vi "Waveform and Laser Controls V7.vi"() -> ()   [LabVIEW 2014]
uses:
  Waveform Scan Parameters.ctl
  <vilib>/Platform/TimedLoop/XDataNode/timing_clust.ctl
  <vilib>/Platform/TimedLoop/XDataNode/nitl_modes.ctl
  <vilib>/Platform/TimedLoop/XDataNode/wakeup.ctl
  <vilib>/rvi/Emulation/niFpgaGetClockAttributes.vi
  <vilib>/rvi/Emulation/niFpgaSctlEmulationGetInTimedLoop.vi
  <vilib>/rvi/Emulation/niFpgaEmulationReportErrorSimple.vi
  <vilib>/rvi/Emulation/niFpgaProcessEmulError.vi
  <vilib>/rvi/eio/common/nirviEmuTemplateMethod_errors.vi
  <vilib>/rvi/Emulation/niFpgaCriticalErrorInLSC.vi
  <vilib>/rvi/Memory/Memory_Emulation/nirvimemoryFastEmulation.vi
  <vilib>/rvi/Memory/Memory_Emulation/nirvimemoryEmulation.vi
  <vilib>/rvi/Emulation/niFpgaEmulationIsFPGAContextNoSignature.vi
  <vilib>/rvi/DataTransferAndStorage/Container/Common/niFpgaContainerGetUniqueNameForEmu.vi
  <vilib>/rvi/errors/nirviReportUnexpectedCaseInternalError (U32).vi
  <vilib>/rvi/Memory/Memory_Emulation/niFpgaMemoryEmulationCacheClearOnFirstRun.vi
  <vilib>/rvi/Memory/Memory_Emulation/nirvimemoryEmulationManagerCache_MakeExclusive.vi
  <vilib>/rvi/Memory/Memory_Emulation/niFpgaMemoryEmulationValidateCache.vi
  <vilib>/rvi/Memory/Memory_Emulation/nirvimemoryEmulationManagerCache_InsertValue.vi
  <vilib>/Utility/error.llb/Clear Errors.vi
  <vilib>/rvi/Memory/Memory_Emulation/nirvimemoryEmulationManagerCache_ReleaseExclusive.vi
  <vilib>/rvi/Memory/Memory_Emulation/nirvimemoryEmulationManagerCache_GetValue.vi
  <vilib>/rvi/Memory/Memory_Emulation/nirvimemoryEmulationManagerCache_SetValue.vi
  <vilib>/eio/EIONode/EIONode.xnode
  <vilib>/rvi/DataTransferAndStorage/Container/XNode/niFpgaContainer.xnode
  <vilib>/Platform/TimedLoop/XDataNode/XDataNode.xnode
  <vilib>/rvi/DataTransferAndStorage/Register/Emulation/niFpgaRegisterEmulation.vi
  <vilib>/Platform/TimedLoop/XDataNode/XDNodeRunTimeDep.lvlib
panel:
  in  "Current Frame":u8
  in  "Lower Shutter Command":bool
  in  "Upper Shutter Command":bool
  out "Lower Shutter Status":bool
  out "Upper Shutter Status":bool
  in  "stop":bool
  in  "775 AOM (I16)":i16=16500
  out "Laser Blank Trigger":bool
  in  "Laser On Time (Ticks)":u8=8
  in  "Sequences":u8=4
  in  "Laser Delay (Ticks)":u8
  in  "Laser States":u32
  in  "Blanking Off/Manual":bool
  in  "Z Piezo Axis":i16
  in  "Y Piezo Axis":i16
  in  "X Piezo Axis":i16
  out "End Linear Ramp":bool
  in  "End of Linear Ramp":u32
  in  "Z Stack Start Position (I16)":i16
  in  "Frames Per Z Step":u8
  in  "Number of Z Steps":u8
  in  "Z Step Size (I16)":i16
  in  "Stop Sync Signal":bool
  in  "Accums Per Line":u32[](array[numeric])=[0, 0, 0, 0]
  in  "Number of Lines":u32
  out "Frame Trigger":bool
  in  "Reset Position Error":bool
  in  "Galvo 1 Position (I16)":i16
  in  "Galvo 2 Position (I16)":i16
  in  "WF 3 Data Loaded":bool
  in  "WF 2 Data Loaded":bool
  in  "Waveform Scan Parameters":T1={"Scanning Mode"=0, "Fast Axis WF Length (Elements)"=0, "Fast Axis Sample Period (Ticks)"=40, "Slow Axis 1 WF Length (Elements)"=0, "Slow Axis 1 Sample Period (Ticks)"=40, "Slow Axis 1 Delay (25 ns) Steps"=40, "Slow Axis 2 WFLength (Elements)"=0, "Slow Axis 2 Sample Period (Ticks)"=40, "Slow Axis 2 Delay (25 ns) Steps"=40}
  in  "Resonant Mirror":T2
  in  "Galvo Mirror 2":T3
  in  "Galvo Mirror 1":T3
  in  "Start Waveforms":bool
  in  "Unused Axis Offset":i16
  in  "Slow Axis 2 Waveform Element":i16
  in  "Fast Axis Waveform Element":i16
  in  "Slow Axis 1 Waveform Element":i16
  in  "WF 1 Data Loaded":bool
  # "V2 - Adding in a line clock\nV3 - Cluster Scan Parameters"
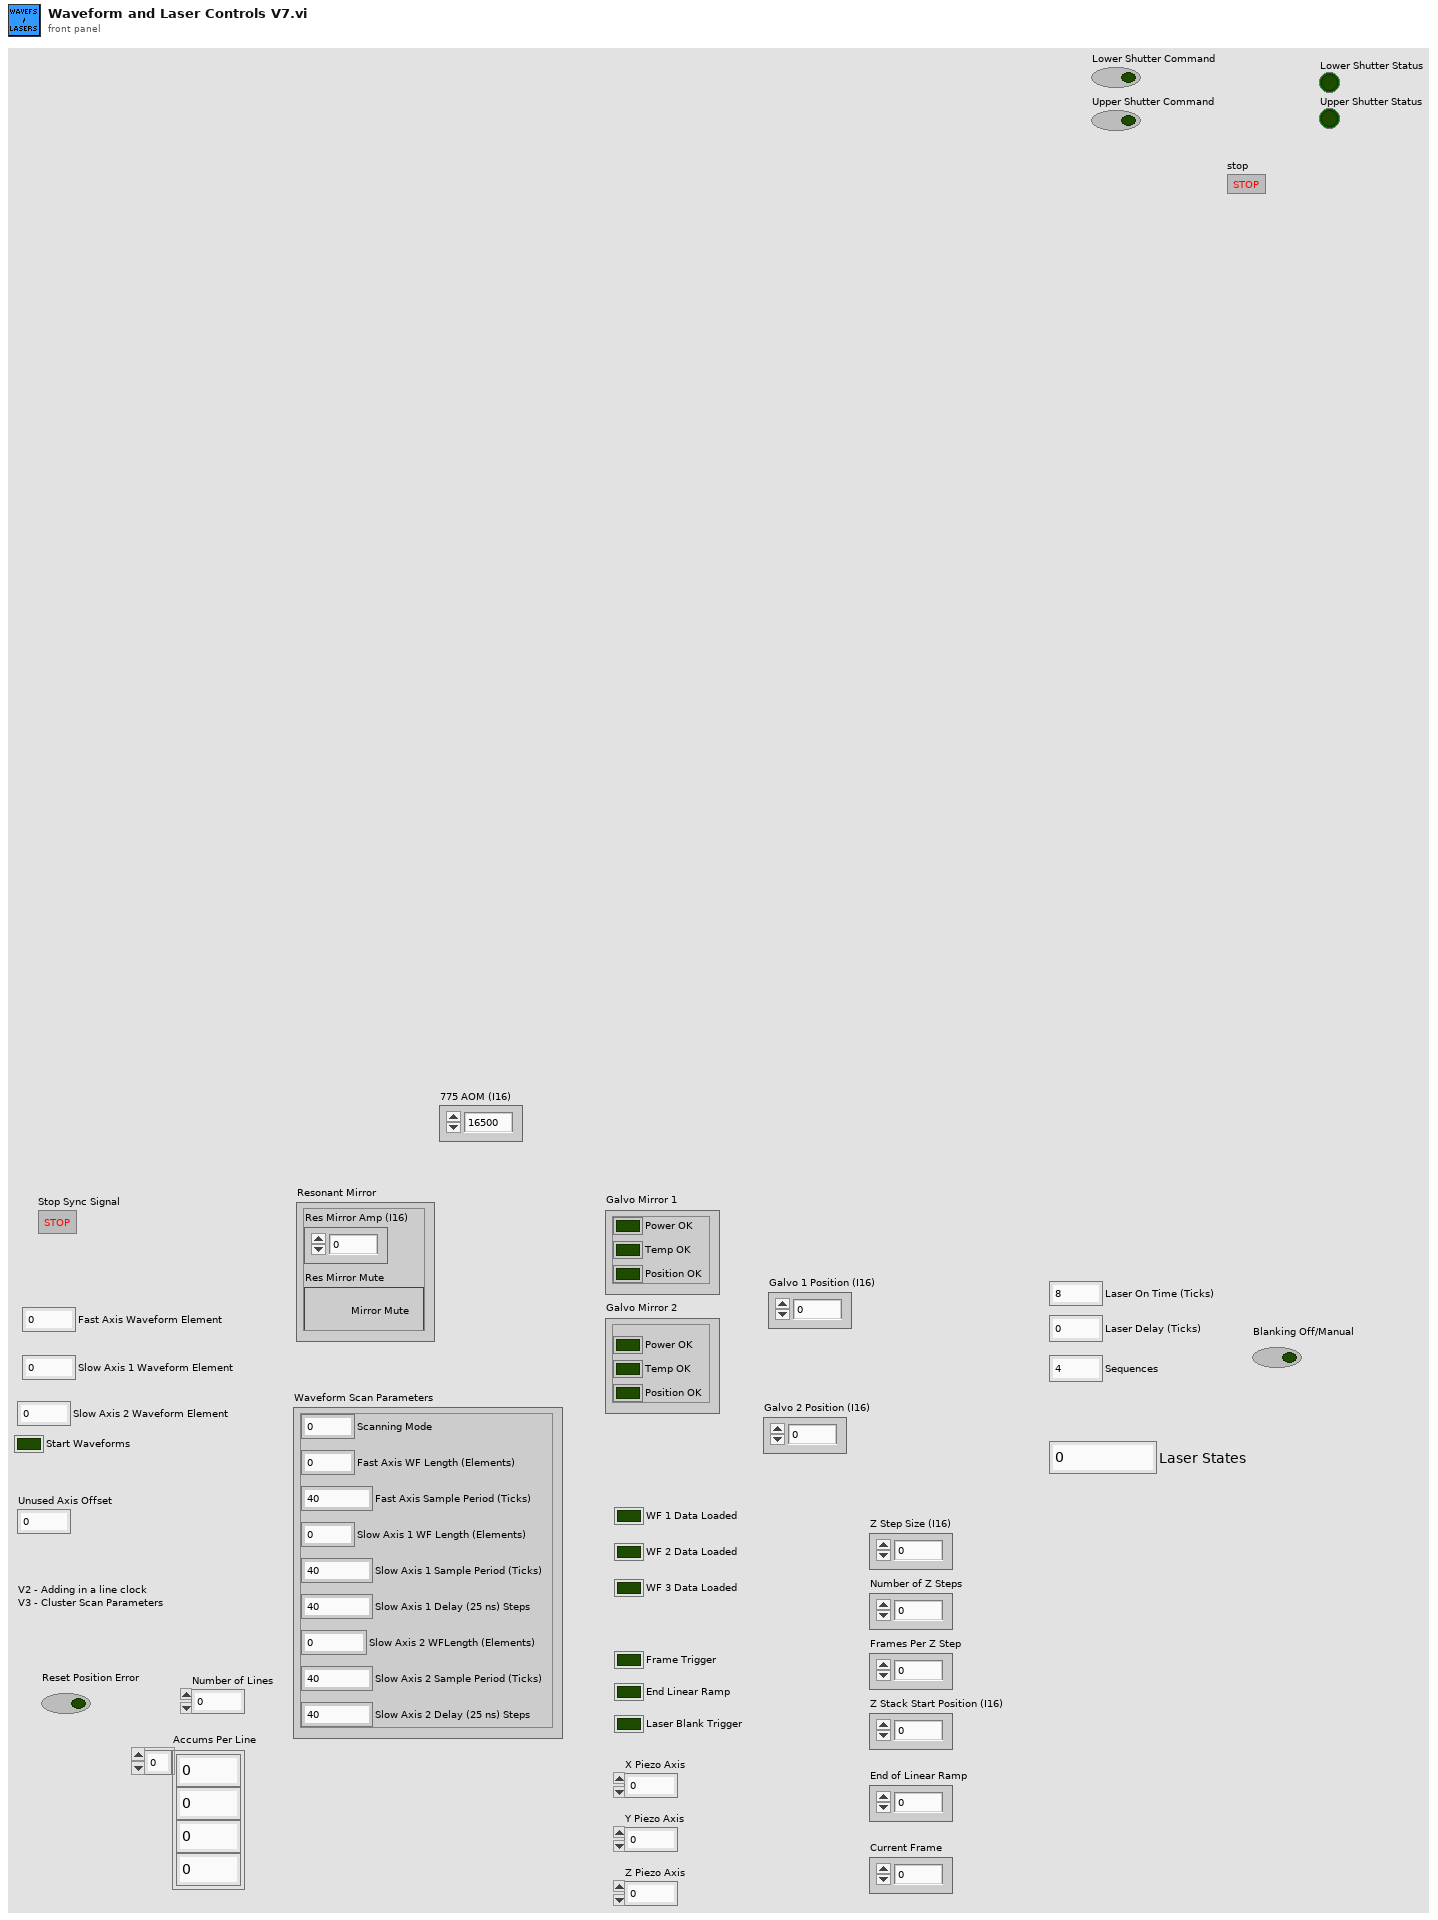
[diagram p1: front panel]
types:
  T1 = typedef "Waveform Scan Parameters.ctl" = cluster{"Scanning Mode":u8, "Fast Axis WF Length (Elements)":i32, "Fast Axis Sample Period (Ticks)":u32, "Slow Axis 1 WF Length (Elements)":i32, "Slow Axis 1 Sample Period (Ticks)":u32, "Slow Axis 1 Delay (25 ns) Steps":i32, "Slow Axis 2 WFLength (Elements)":i32, "Slow Axis 2 Sample Period (Ticks)":u32, "Slow Axis 2 Delay (25 ns) Steps":i32}
  T2 = cluster{"Res Mirror Amp (I16)":i16, "Res Mirror Mute":bool}
  T3 = cluster{"Power OK":bool, "Temp OK":bool, "Position OK":bool}
  T4 = typedef "XDNodeRunTimeDep.lvlib/timing_clust.ctl" = cluster{"Expected End [f-1]":u64, "Actual End [f-1]":u64, "Finished Late? [f-1]":bool, "Expected End [i-1]":u64, "Actual End [i-1]":u64, "Finished Late? [i-1]":bool, "Expected Start [i]":u64, "Actual Start [i]":u64, "Expected Start [f]":u64, "Actual Start [f]":u64, "Source Name":string, "Structure Name":string, "Period":i64, "Deadline":i64, "Offset":i64, "Start":i64, "Priority":i32, "Timeout":i32, "Mode":T5, "Wakeup Reason":T6, "Error":errorcluster, "Source Type":string, "Secondary Source Type":string, "Global End Time":u64, "Global Start Time":u64, "Frame Duration":u64, "Iteration Duration":u64, "Assigned CPU":i32, "I/O Scan Engine Mode":u32}
  T5 = typedef "XDNodeRunTimeDep.lvlib/nitl_modes.ctl" = enum32{"No Change", "Process missed periods, maintain original phase", "Discard missed periods, maintain original phase", "Process missed periods, ignore original phase", "Discard missed periods, ignore original phase"}
  T6 = typedef "XDNodeRunTimeDep.lvlib/wakeup.ctl" = enum32{"Normal", "Aborted", "Asynchronous wakeup", "Timing source error", "Timed loop error", "Timeout"}
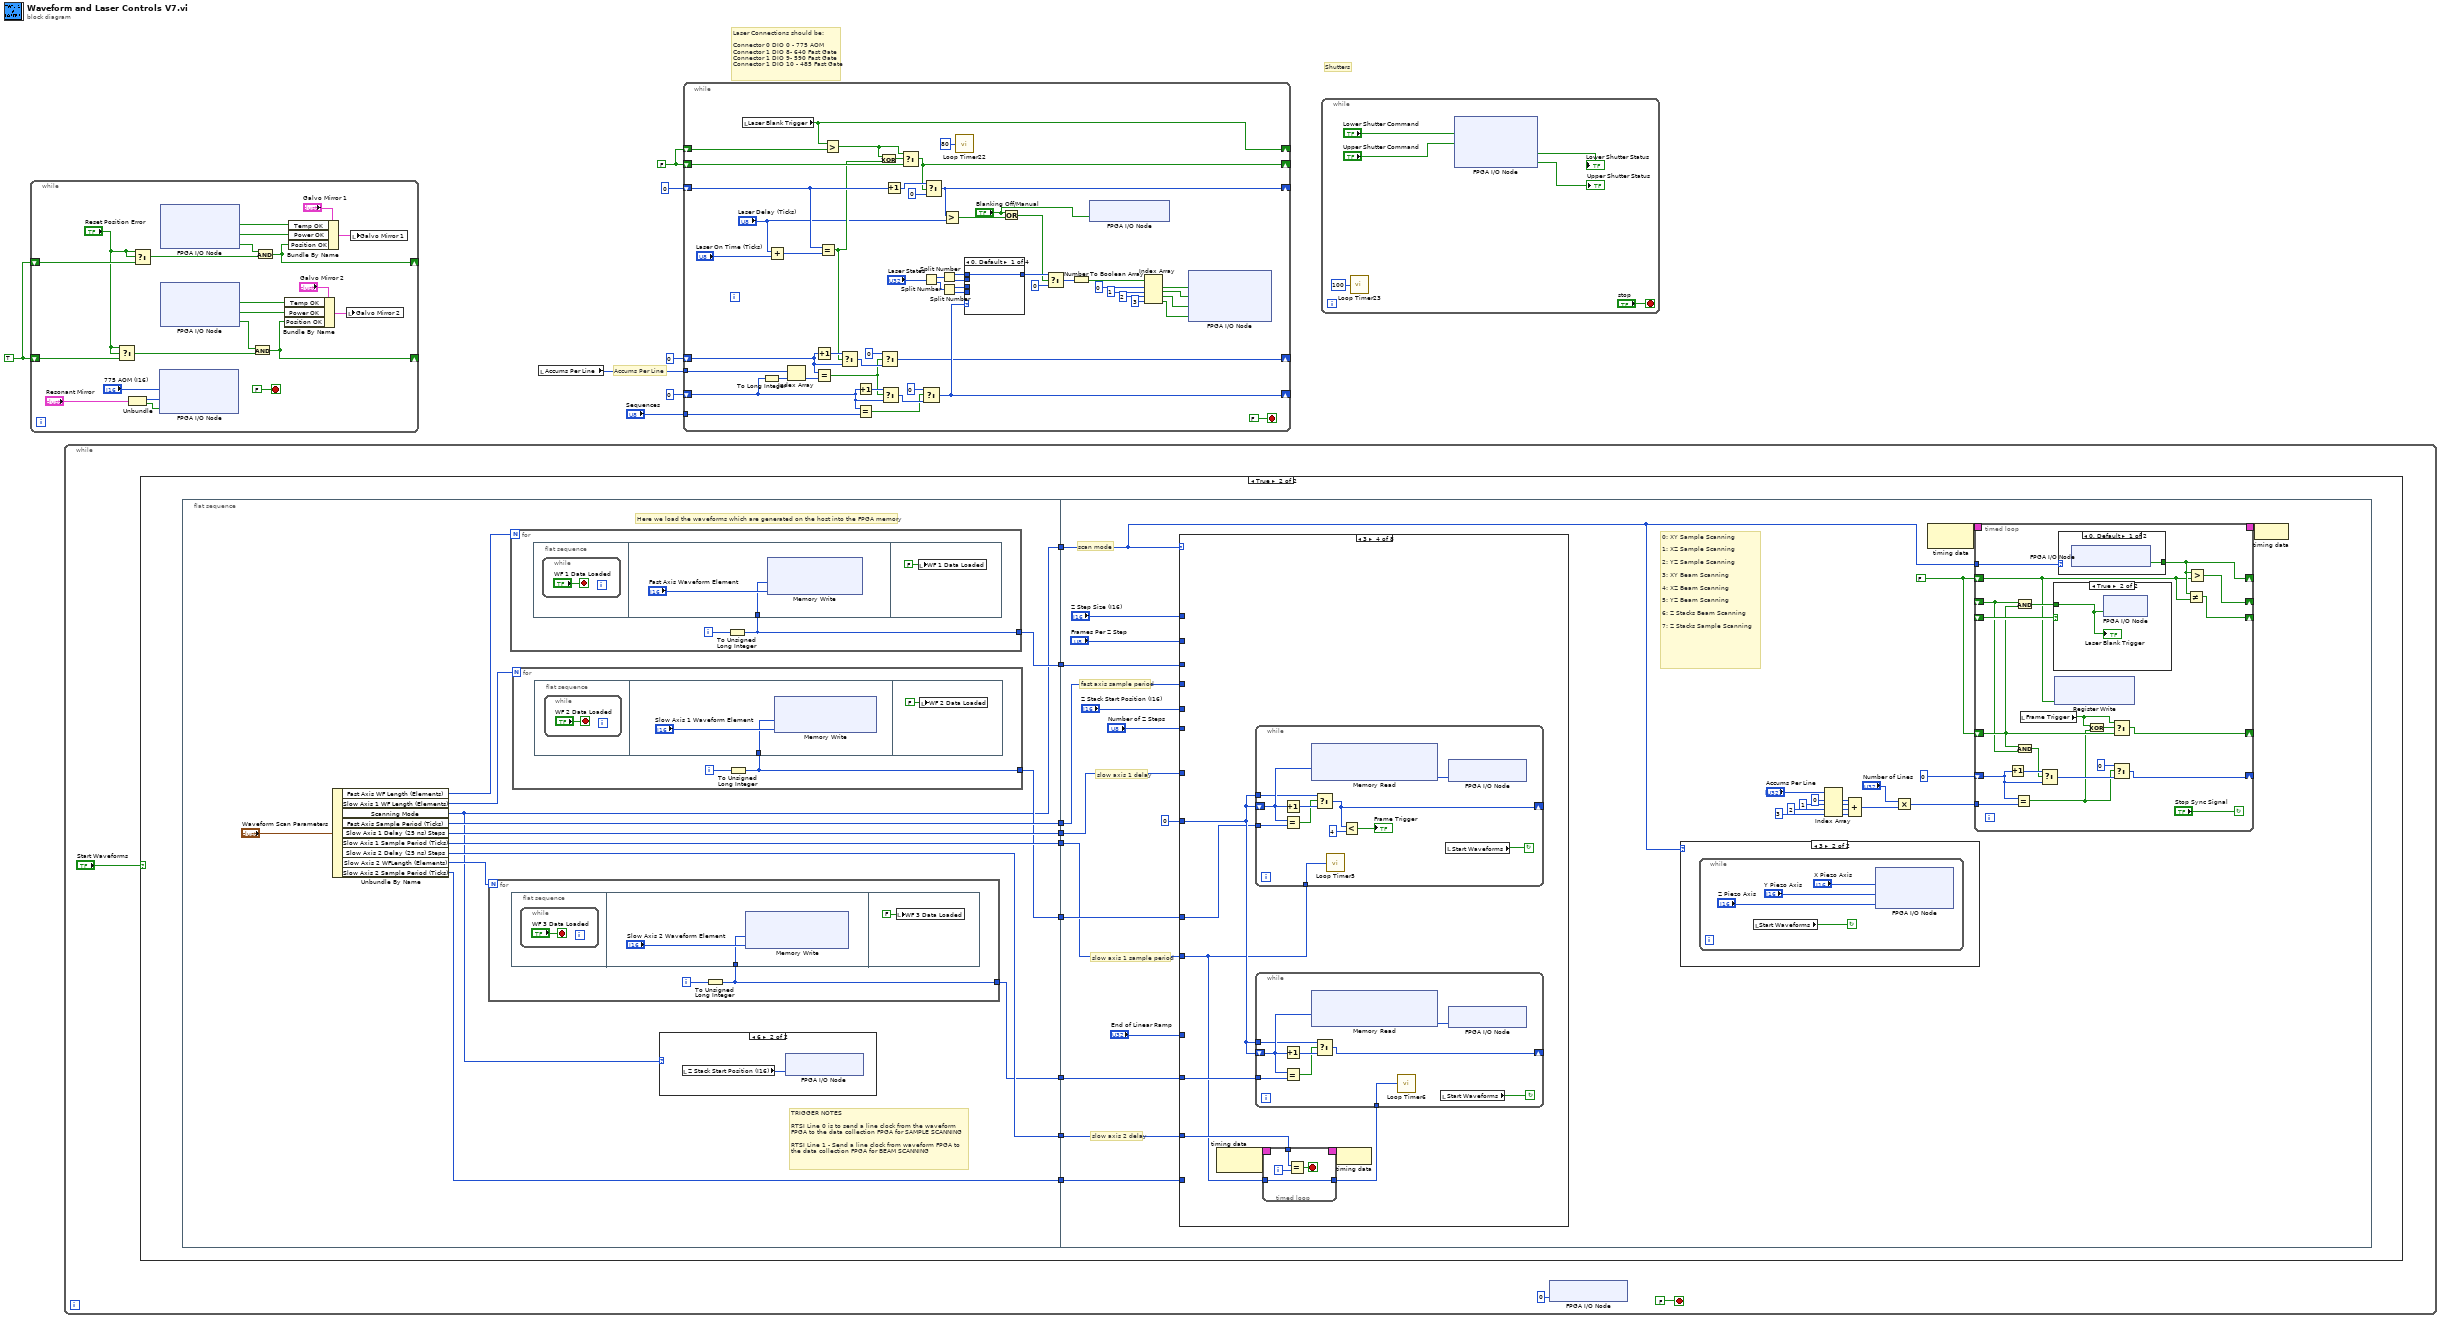
[diagram p0: block diagram]
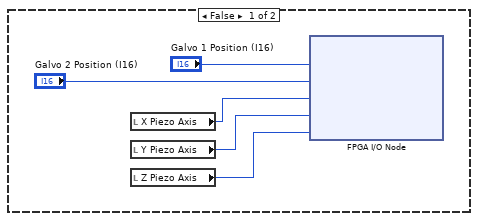
[diagram p5: hidden frame]
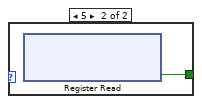
[diagram p7: hidden frame]
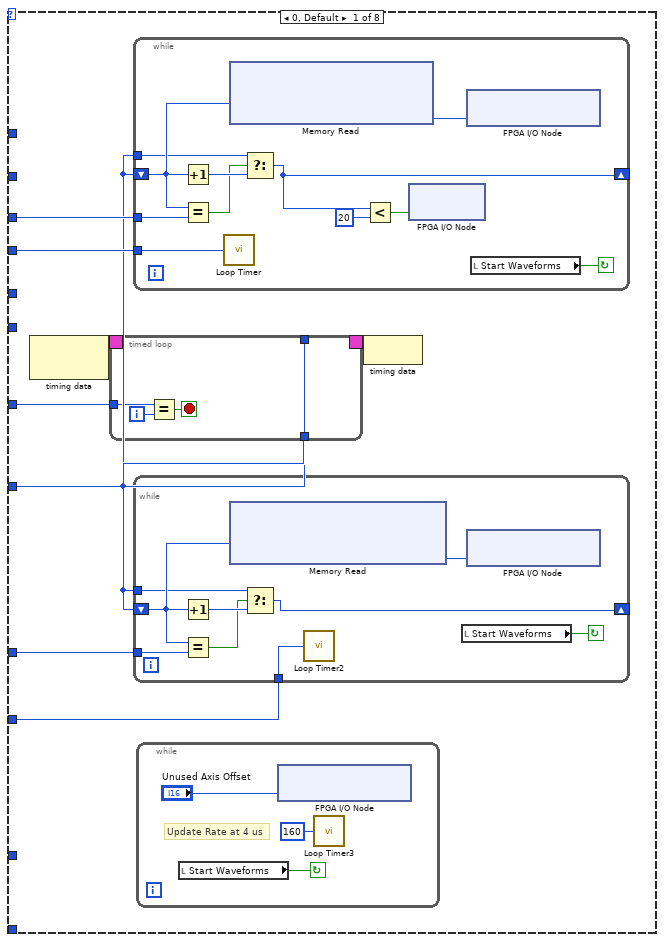
[diagram p10: hidden frame]
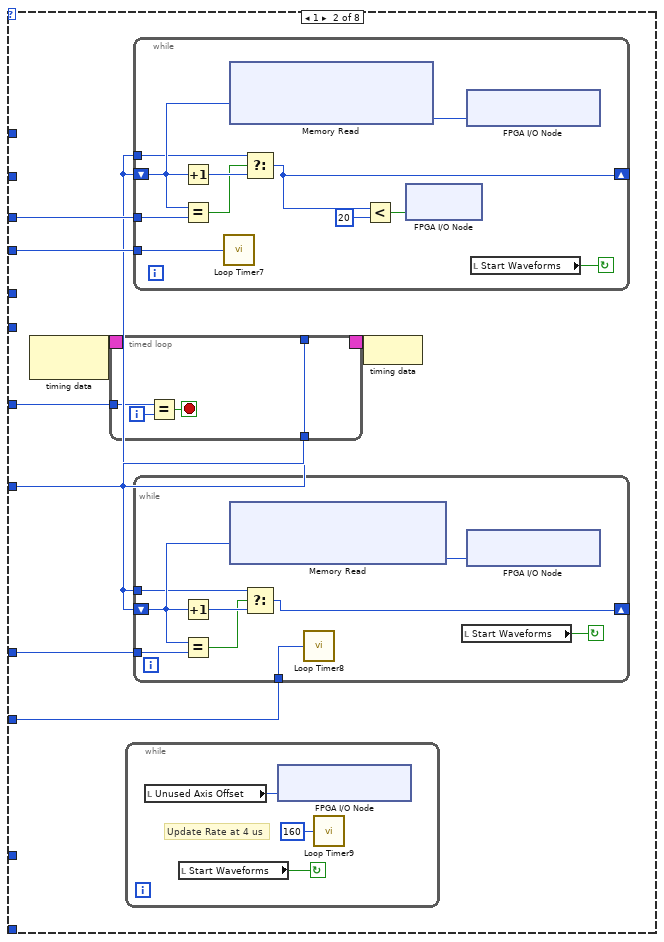
[diagram p11: hidden frame]
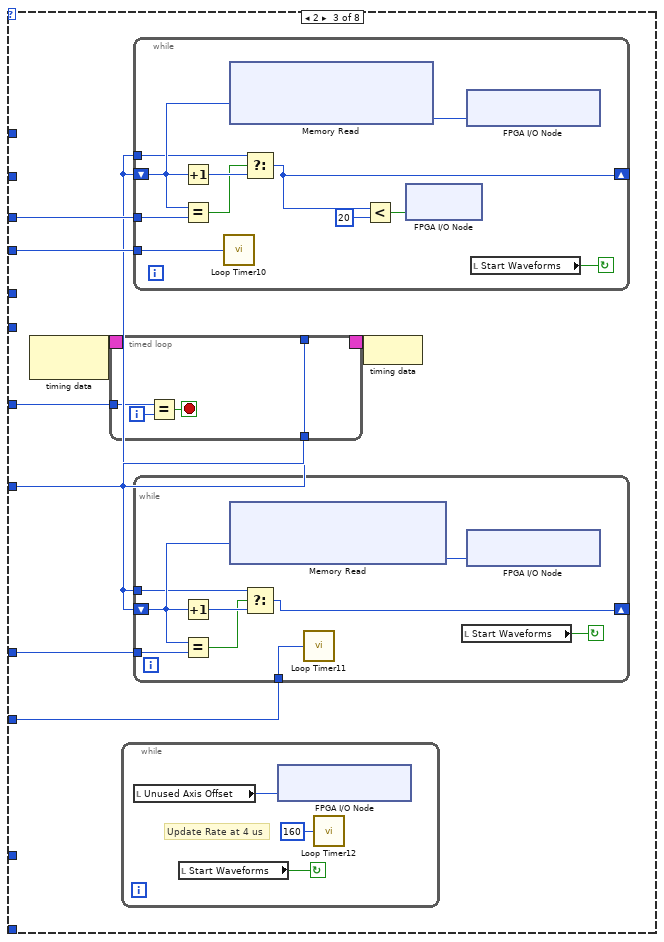
[diagram p12: hidden frame]
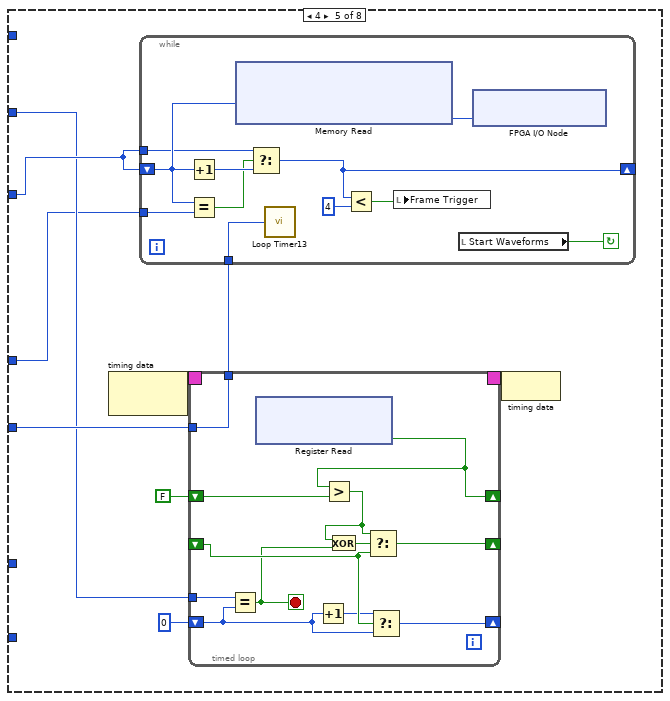
[diagram p13: hidden frame]
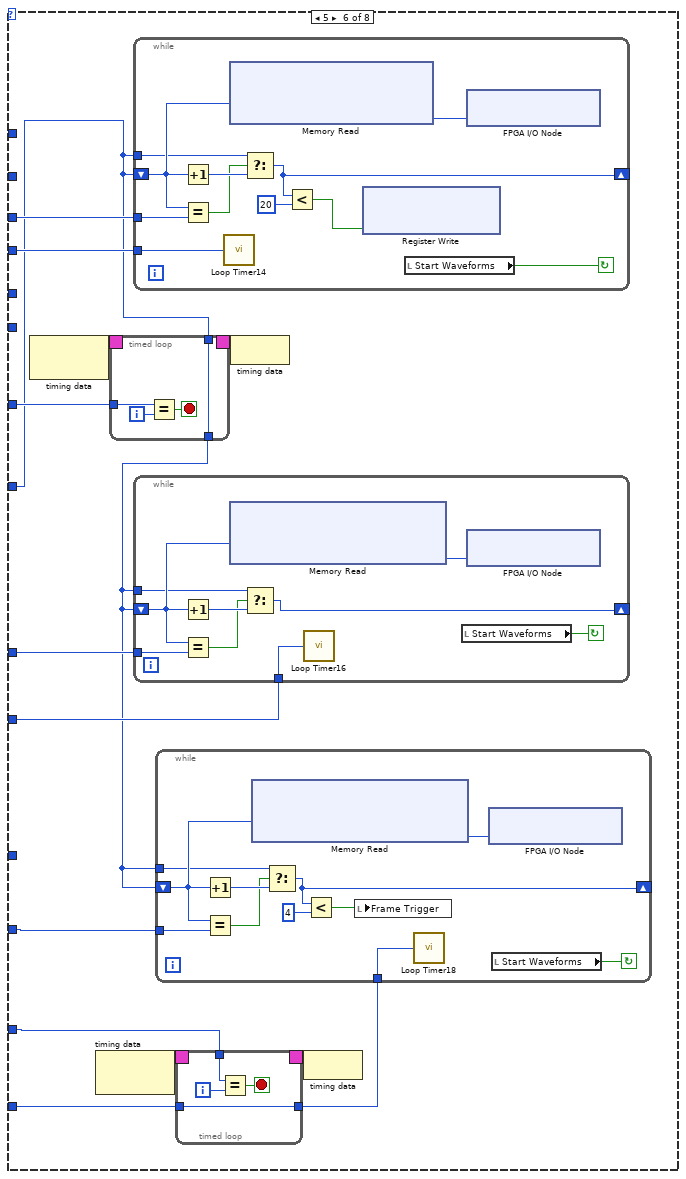
[diagram p14: hidden frame]
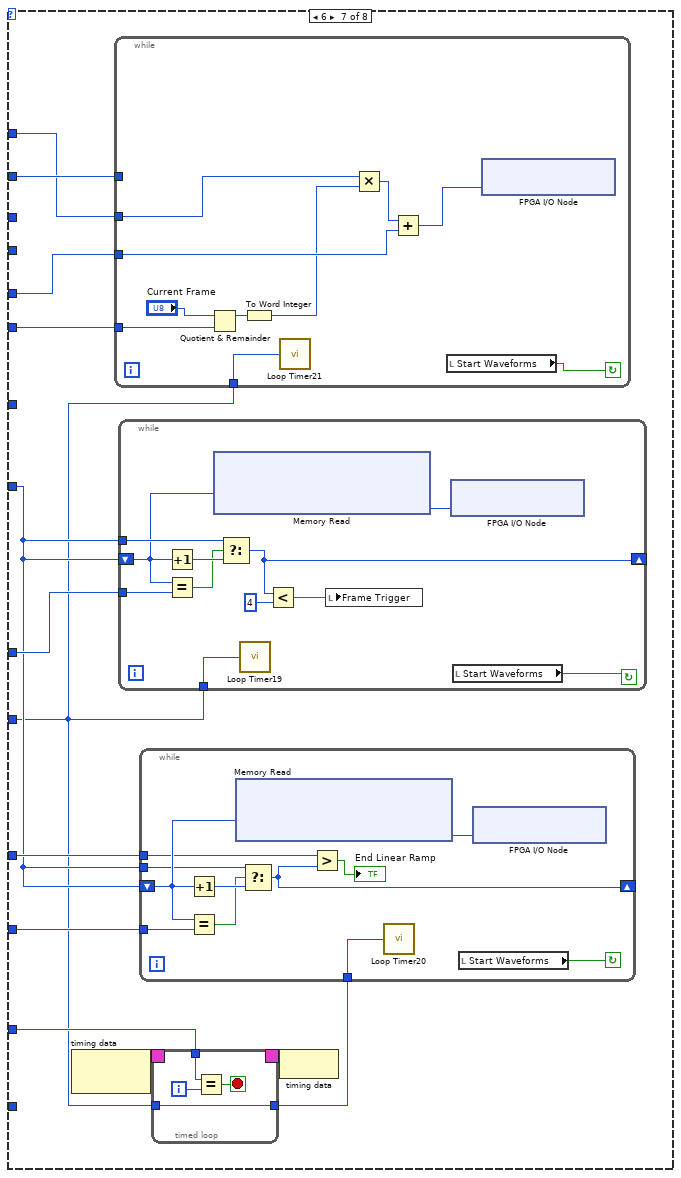
[diagram p15: hidden frame]
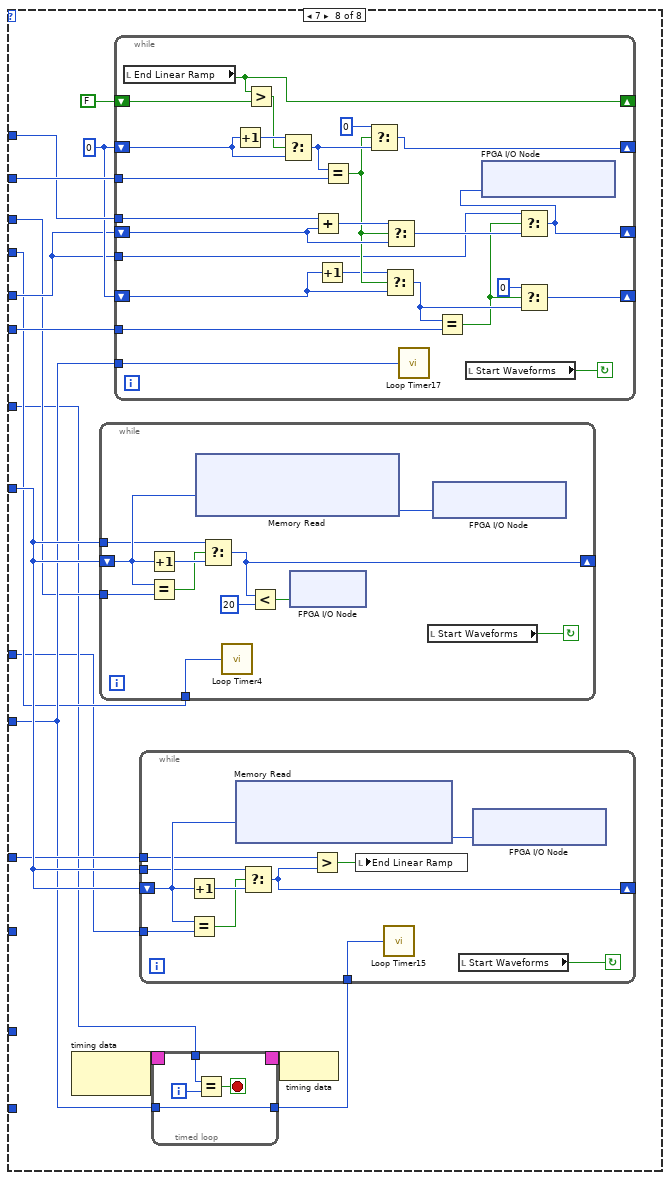
[diagram p16: hidden frame]
diagram:
  w2 = FALSE
  w7 = TRUE
  # "Shutters"
  # "Laser Connections should be:\n\nConnector 0 DIO 0 - 775 AOM\nConnector 1 DIO 8- 640 Fast Gate\nConnector 1 DIO 9- 590 Fast Gate\nConnector 1 DIO 10 - 485 Fast Gate"
  # "Accums Per Line"
  n1 = while {
    shift-right: [w15] -> _
    shift-left: w7 -> [w17]
    shift-right: [w11] -> _
    shift-left: w7 -> [w13]
    stop <- FALSE stop-if-true
    n2 = Select(t="Reset Position Error", s="Reset Position Error", f=w17) -> (s? t:f=w16:bool)
    n3 = Unbundle("Resonant Mirror") -> ("Res Mirror Amp (I16)"=w27:i16, "Res Mirror Mute"=w26:bool)
    n4 = Select(t="Reset Position Error", s="Reset Position Error", f=w13) -> (s? t:f=w12:bool)
    n5 = xnode "FPGA I/O Node"("Connector0/AO4"="775 AOM (I16)", "Connector0/AO7"=w27, "Connector0/DIO7"=w26) -> ()  [unwired: 4 in, 4 out]
    n6 = xnode "FPGA I/O Node"() -> ("Connector0/DIO1"=w8:bool, "Connector0/DIO2"=w25:bool, "Connector0/DIO3"=w14:bool)  [unwired: 4 in, 4 out]
    n7 = xnode "FPGA I/O Node"() -> ("Connector0/DIO4"=w19:bool, "Connector0/DIO5"=w20:bool, "Connector0/DIO6"=w18:bool)  [unwired: 4 in, 4 out]
    n8 = And(x=w18, y=w16) -> (x .and. y?=w15:bool)
    n9 = And(x=w14, y=w12) -> (x .and. y?=w11:bool)
    n10 = Bundle By Name(cluster="Galvo Mirror 2", "Temp OK"=w19, "Power OK"=w20, "Position OK"=w15) -> (w22:T3)
    n11 = Bundle By Name(cluster="Galvo Mirror 1", "Temp OK"=w8, "Power OK"=w25, "Position OK"=w11) -> (w24:T3)
    n12 = local write "Galvo Mirror 2"(w22) -> ()
    n13 = local write "Galvo Mirror 1"(w24) -> ()
  }
  n14 = while {
    stop <- FALSE stop-if-true
    n15 = case shown="True" "Start Waveforms" {
      frame False {
        n16 = local read "X Piezo Axis"() -> (w35:i16)
        n17 = local read "Y Piezo Axis"() -> (w34:i16)
        n18 = local read "Z Piezo Axis"() -> (w33:i16)
        n19 = xnode "FPGA I/O Node"("Connector0/AO5"="Galvo 1 Position (I16)", "Connector0/AO6"="Galvo 2 Position (I16)", "Connector0/AO1"=w35, "Connector0/AO2"=w34, "Connector0/AO3"=w33) -> ()  [unwired: 5 in, 5 out]
      }
      frame True {
        n20 = flat-sequence {
          tunnel: [w59] -> w46
          tunnel: [w49] -> w45
          tunnel: [w50] -> w44
          tunnel: [w48] -> w43
          tunnel: [w57] -> w42
          tunnel: [w56] -> w41
          tunnel: [w55] -> w40
          tunnel: [w54] -> w39
          tunnel: [w47] -> w38
          tunnel: w46 -> [w109]
          tunnel: w45 -> [w108]
          tunnel: w44 -> [w106]
          tunnel: w43 -> [w80]
          tunnel: w42 -> [w105]
          tunnel: w41 -> [w104]
          tunnel: w40 -> [w103]
          tunnel: w39 -> [w102]
          tunnel: w38 -> [w79]
          frame #0 {
            # "TRIGGER NOTES\n\nRTSI Line 0 is to send a line clock from the waveform\nFPGA to the data collection FPGA for SAMPLE SCANNING\n\nRTSI Line 1 - Send a line clock from waveform FPGA to\nthe data collection FPGA for BEAM SCANNING"
            # "Here we load the waveforms which are generated on the host into the FPGA memory"
            n21 = Unbundle By Name("Waveform Scan Parameters") -> ("Fast Axis WF Length (Elements)"=w53:i32, "Slow Axis 1 WF Length (Elements)"=w52:i32, "Scanning Mode"=w48:u8, "Fast Axis Sample Period (Ticks)"=w57:u32, "Slow Axis 1 Delay (25 ns) Steps"=w56:i32, "Slow Axis 1 Sample Period (Ticks)"=w55:u32, "Slow Axis 2 Delay (25 ns) Steps"=w54:i32, "Slow Axis 2 WFLength (Elements)"=w51:i32, "Slow Axis 2 Sample Period (Ticks)"=w47:u32)
            n22 = for {
              N: w51 -> [_]
              tunnel: [w61] -> w49
              i -> [w62]
              n23 = flat-sequence {
                tunnel: w61 -> [w64]
                frame #0 {
                  n24 = while {
                    stop <- "WF 3 Data Loaded" stop-if-true
                  }
                }
                frame #1 {
                  n25 = xnode ("Memory Write")("Address"=w64, "Data"="Slow Axis 2 Waveform Element") -> ()  [unwired: 1 in, 1 out]
                }
                frame #2 {
                  n26 = local write "WF 3 Data Loaded"(FALSE ("Host Data Loaded")) -> ()
                }
              }
              n27 = To Unsigned Long Integer(number=w62) -> (unsigned 32bit integer=w61:u32)
            }
            n28 = for {
              N: w53 -> [_]
              tunnel: [w73] -> w59
              i -> [w74]
              n29 = flat-sequence {
                tunnel: w73 -> [w76]
                frame #0 {
                  n30 = while {
                    stop <- "WF 1 Data Loaded" stop-if-true
                  }
                }
                frame #1 {
                  n31 = xnode ("Memory Write")("Address"=w76, "Data"="Fast Axis Waveform Element") -> ()  [unwired: 1 in, 1 out]
                }
                frame #2 {
                  n32 = local write "WF 1 Data Loaded"(FALSE ("Host Data Loaded")) -> ()
                }
              }
              n33 = To Unsigned Long Integer(number=w74) -> (unsigned 32bit integer=w73:u32)
            }
            n34 = for {
              N: w52 -> [_]
              tunnel: [w67] -> w50
              i -> [w68]
              n35 = flat-sequence {
                tunnel: w67 -> [w70]
                frame #0 {
                  n36 = while {
                    stop <- "WF 2 Data Loaded" stop-if-true
                  }
                }
                frame #1 {
                  n37 = xnode ("Memory Write")("Address"=w70, "Data"="Slow Axis 1 Waveform Element") -> ()  [unwired: 1 in, 1 out]
                }
                frame #2 {
                  n38 = local write "WF 2 Data Loaded"(FALSE ("Host Data Loaded")) -> ()
                }
              }
              n39 = To Unsigned Long Integer(number=w68) -> (unsigned 32bit integer=w67:u32)
            }
            n40 = case shown="6" w48 {
              frame 0, Default {
              }
              frame 6 {
                n41 = local read "Z Stack Start Position (I16)"() -> (w60:i16)
                n42 = xnode "FPGA I/O Node"("Connector0/AO3"=w60) -> ()  [unwired: 1 in, 1 out]
              }
            }
          }
          frame #1 {
            w82 = FALSE
            # "slow axis 2 delay"
            # "slow axis 1 sample period"
            # "slow axis 1 delay"
            # "fast axis sample period"
            # "scan mode"
            # "0: XY Sample Scanning\n\n1: XZ Sample Scanning\n\n2: YZ Sample Scanning\n\n3: XY Beam Scanning\n\n4: XZ Beam Scanning\n\n5: YZ Beam Scanning\n\n6: Z Stacks Beam Scanning\n\n7: Z Stacks Sample Scanning"
            n43 = case shown="3" w80 {
              tunnel: w109 -> [w148 w188 w228 _ _ w348 _ w451]
              tunnel: w105 -> [w147 w187 w227 _ _ w347 _ w452]
              tunnel: w108 -> [_ _ _ w269 _ w342 w408 _]
              tunnel: u32 0 -> [w142 w182 w222 w268 w306 w344 w398 w464]
              tunnel: w104 -> [w146 w186 w226 _ w304 w346 _ w450]
              tunnel: w102 -> [_ _ _ w267 _ w341 w407 _]
              tunnel: w106 -> [w144 w184 w224 w262 w303 w345 w404 w449]
              tunnel: w103 -> [w143 w183 w223 w263 w305 w343 w396 w453]
              tunnel: "Frames Per Z Step" -> [_ _ _ _ _ _ w403 w460]
              tunnel: "Z Stack Start Position (I16)" -> [_ _ _ _ _ _ w399 w456]
              tunnel: "Z Step Size (I16)" -> [_ _ _ _ _ _ w402 w459]
              tunnel: "Number of Z Steps" -> [_ _ _ _ _ _ w401 w457]
              tunnel: "End of Linear Ramp" -> [_ _ _ _ _ _ w400 w455]
              tunnel: w79 -> [_ _ _ _ _ w334 _ _]
              frame 0, Default {
                n44 = node-c288() -> (w150:T4)  [unwired: 1 in]
                n45 = timed-loop {
                  timing: w150 -> [_]
                  timing-out: [_] -> w149
                  tunnel: w146 -> [w155]
                  tunnel: w142 -> [w154]
                  tunnel: [w154] -> w145
                  i -> [w157]
                  stop <- w156 stop-if-true
                  n46 = Equal?(x=w155, y=w157) -> (x = y?=w156:bool)
                }
                n47 = while {
                  shift-right: [w173] -> _
                  shift-left: w142 -> [w179]
                  tunnel: w148 -> [w180]
                  tunnel: w147 -> [w177]
                  tunnel: w142 -> [w176]
                  stop <- w175 continue-if-true
                  n48 = Increment(x=w179) -> (x+1=w181:u32)
                  n49 = Equal?(x=w179, y=w180) -> (x = y?=w174:bool)
                  n50 = call "Loop Timer"("Count(Ticks)"=w177) -> ()  [unwired: 1 out]
                  n51 = xnode ("Memory Read")("Address"=w179) -> ("Data"=w178:i16)  [unwired: 1 in, 1 out]
                  n52 = Select(t=w176, s=w174, f=w181) -> (s? t:f=w173:u32)
                  n53 = Less?(x=w173, y=u32 20) -> (x < y?=w171:bool)
                  n54 = xnode "FPGA I/O Node"("TRIG0"=w171) -> ()  [unwired: 1 in, 1 out]
                  n55 = xnode "FPGA I/O Node"("Connector0/AO1"=w178) -> ()  [unwired: 1 in, 1 out]
                  n56 = local read "Start Waveforms"() -> (w175:bool)
                }
                n57 = while {
                  shift-right: [w169] -> _
                  shift-left: w145 -> [w166]
                  tunnel: w144 -> [w168]
                  tunnel: w145 -> [w164]
                  tunnel: w143 -> [w163]
                  stop <- w162 continue-if-true
                  n58 = Increment(x=w166) -> (x+1=w170:u32)
                  n59 = Equal?(x=w166, y=w168) -> (x = y?=w167:bool)
                  n60 = xnode ("Memory Read")("Address"=w166) -> ("Data"=w165:i16)  [unwired: 1 in, 1 out]
                  n61 = Select(t=w164, s=w167, f=w170) -> (s? t:f=w169:u32)
                  n62 = call "Loop Timer2"("Count(Ticks)"=w163) -> ()  [unwired: 1 out]
                  n63 = local read "Start Waveforms"() -> (w162:bool)
                  n64 = xnode "FPGA I/O Node"("Connector0/AO2"=w165) -> ()  [unwired: 1 in, 1 out]
                }
                n65 = while {
                  stop <- w151 continue-if-true
                  # "Update Rate at 4 us"
                  n66 = local read "Start Waveforms"() -> (w151:bool)
                  n67 = xnode "FPGA I/O Node"("Connector0/AO3"="Unused Axis Offset") -> ()  [unwired: 1 in, 1 out]
                  n68 = call "Loop Timer3"("Count(Ticks)"=u32 160) -> ()  [unwired: 1 out]
                }
                n69 = node-c288(w149) -> ()
              }
              frame 1 {
                n70 = node-c288() -> (w190:T4)  [unwired: 1 in]
                n71 = timed-loop {
                  timing: w190 -> [_]
                  timing-out: [_] -> w189
                  tunnel: w186 -> [w195]
                  tunnel: w182 -> [w194]
                  tunnel: [w194] -> w185
                  i -> [w197]
                  stop <- w196 stop-if-true
                  n72 = Equal?(x=w195, y=w197) -> (x = y?=w196:bool)
                }
                n73 = while {
                  stop <- w192 continue-if-true
                  # "Update Rate at 4 us"
                  n74 = local read "Unused Axis Offset"() -> (w191:i16)
                  n75 = local read "Start Waveforms"() -> (w192:bool)
                  n76 = xnode "FPGA I/O Node"("Connector0/AO2"=w191) -> ()  [unwired: 1 in, 1 out]
                  n77 = call "Loop Timer9"("Count(Ticks)"=u32 160) -> ()  [unwired: 1 out]
                }
                n78 = while {
                  shift-right: [w213] -> _
                  shift-left: w182 -> [w219]
                  tunnel: w188 -> [w220]
                  tunnel: w187 -> [w217]
                  tunnel: w182 -> [w216]
                  stop <- w215 continue-if-true
                  n79 = Increment(x=w219) -> (x+1=w221:u32)
                  n80 = Equal?(x=w219, y=w220) -> (x = y?=w214:bool)
                  n81 = call "Loop Timer7"("Count(Ticks)"=w217) -> ()  [unwired: 1 out]
                  n82 = xnode ("Memory Read")("Address"=w219) -> ("Data"=w218:i16)  [unwired: 1 in, 1 out]
                  n83 = Select(t=w216, s=w214, f=w221) -> (s? t:f=w213:u32)
                  n84 = Less?(x=w213, y=u32 20) -> (x < y?=w211:bool)
                  n85 = xnode "FPGA I/O Node"("TRIG0"=w211) -> ()  [unwired: 1 in, 1 out]
                  n86 = xnode "FPGA I/O Node"("Connector0/AO1"=w218) -> ()  [unwired: 1 in, 1 out]
                  n87 = local read "Start Waveforms"() -> (w215:bool)
                }
                n88 = while {
                  shift-right: [w209] -> _
                  shift-left: w185 -> [w206]
                  tunnel: w184 -> [w208]
                  tunnel: w185 -> [w204]
                  tunnel: w183 -> [w203]
                  stop <- w202 continue-if-true
                  n89 = Increment(x=w206) -> (x+1=w210:u32)
                  n90 = Equal?(x=w206, y=w208) -> (x = y?=w207:bool)
                  n91 = xnode ("Memory Read")("Address"=w206) -> ("Data"=w205:i16)  [unwired: 1 in, 1 out]
                  n92 = Select(t=w204, s=w207, f=w210) -> (s? t:f=w209:u32)
                  n93 = call "Loop Timer8"("Count(Ticks)"=w203) -> ()  [unwired: 1 out]
                  n94 = local read "Start Waveforms"() -> (w202:bool)
                  n95 = xnode "FPGA I/O Node"("Connector0/AO3"=w205) -> ()  [unwired: 1 in, 1 out]
                }
                n96 = node-c288(w189) -> ()
              }
              frame 2 {
                n97 = node-c288() -> (w230:T4)  [unwired: 1 in]
                n98 = timed-loop {
                  timing: w230 -> [_]
                  timing-out: [_] -> w229
                  tunnel: w226 -> [w235]
                  tunnel: w222 -> [w234]
                  tunnel: [w234] -> w225
                  i -> [w237]
                  stop <- w236 stop-if-true
                  n99 = Equal?(x=w235, y=w237) -> (x = y?=w236:bool)
                }
                n100 = while {
                  stop <- w232 continue-if-true
                  # "Update Rate at 4 us"
                  n101 = local read "Unused Axis Offset"() -> (w231:i16)
                  n102 = local read "Start Waveforms"() -> (w232:bool)
                  n103 = xnode "FPGA I/O Node"("Connector0/AO1"=w231) -> ()  [unwired: 1 in, 1 out]
                  n104 = call "Loop Timer12"("Count(Ticks)"=u32 160) -> ()  [unwired: 1 out]
                }
                n105 = while {
                  shift-right: [w253] -> _
                  shift-left: w222 -> [w259]
                  tunnel: w228 -> [w260]
                  tunnel: w227 -> [w257]
                  tunnel: w222 -> [w256]
                  stop <- w255 continue-if-true
                  n106 = Increment(x=w259) -> (x+1=w261:u32)
                  n107 = Equal?(x=w259, y=w260) -> (x = y?=w254:bool)
                  n108 = call "Loop Timer10"("Count(Ticks)"=w257) -> ()  [unwired: 1 out]
                  n109 = xnode ("Memory Read")("Address"=w259) -> ("Data"=w258:i16)  [unwired: 1 in, 1 out]
                  n110 = Select(t=w256, s=w254, f=w261) -> (s? t:f=w253:u32)
                  n111 = Less?(x=w253, y=u32 20) -> (x < y?=w251:bool)
                  n112 = xnode "FPGA I/O Node"("TRIG0"=w251) -> ()  [unwired: 1 in, 1 out]
                  n113 = xnode "FPGA I/O Node"("Connector0/AO2"=w258) -> ()  [unwired: 1 in, 1 out]
                  n114 = local read "Start Waveforms"() -> (w255:bool)
                }
                n115 = while {
                  shift-right: [w249] -> _
                  shift-left: w225 -> [w246]
                  tunnel: w224 -> [w248]
                  tunnel: w225 -> [w244]
                  tunnel: w223 -> [w243]
                  stop <- w242 continue-if-true
                  n116 = Increment(x=w246) -> (x+1=w250:u32)
                  n117 = Equal?(x=w246, y=w248) -> (x = y?=w247:bool)
                  n118 = xnode ("Memory Read")("Address"=w246) -> ("Data"=w245:i16)  [unwired: 1 in, 1 out]
                  n119 = Select(t=w244, s=w247, f=w250) -> (s? t:f=w249:u32)
                  n120 = call "Loop Timer11"("Count(Ticks)"=w243) -> ()  [unwired: 1 out]
                  n121 = local read "Start Waveforms"() -> (w242:bool)
                  n122 = xnode "FPGA I/O Node"("Connector0/AO3"=w245) -> ()  [unwired: 1 in, 1 out]
                }
                n123 = node-c288(w229) -> ()
              }
              frame 3 {
                n124 = node-c288() -> (w266:T4)  [unwired: 1 in]
                n125 = while {
                  shift-right: [w289] -> _
                  shift-left: w268 -> [w295]
                  tunnel: w262 -> [w296]
                  tunnel: w263 -> [w293]
                  tunnel: w268 -> [w292]
                  stop <- w291 continue-if-true
                  n126 = Increment(x=w295) -> (x+1=w297:u32)
                  n127 = Equal?(x=w295, y=w296) -> (x = y?=w290:bool)
                  n128 = xnode ("Memory Read")("Address"=w295) -> ("Data"=w294:i16)  [unwired: 1 in, 1 out]
                  n129 = Select(t=w292, s=w290, f=w297) -> (s? t:f=w289:u32)
                  n130 = call "Loop Timer5"("Count(Ticks)"=w293) -> ()  [unwired: 1 out]
                  n131 = Less?(x=w289, y=u32 4) -> (x < y?=→"Frame Trigger":bool)
                  n132 = local read "Start Waveforms"() -> (w291:bool)
                  n133 = xnode "FPGA I/O Node"("Connector0/AO5"=w294) -> ()  [unwired: 1 in, 1 out]
                }
                n134 = timed-loop {
                  timing: w266 -> [_]
                  timing-out: [_] -> w265
                  tunnel: w263 -> [w279]
                  tunnel: [w279] -> w264
                  tunnel: w267 -> [w280]
                  i -> [w282]
                  stop <- w281 stop-if-true
                  n135 = Equal?(x=w280, y=w282) -> (x = y?=w281:bool)
                }
                n136 = while {
                  shift-right: [w277] -> _
                  shift-left: w268 -> [w275]
                  tunnel: w269 -> [w276]
                  tunnel: w264 -> [w273]
                  tunnel: w268 -> [w272]
                  stop <- w271 continue-if-true
                  n137 = Increment(x=w275) -> (x+1=w278:u32)
                  n138 = Equal?(x=w275, y=w276) -> (x = y?=w270:bool)
                  n139 = xnode ("Memory Read")("Address"=w275) -> ("Data"=w274:i16)  [unwired: 1 in, 1 out]
                  n140 = Select(t=w272, s=w270, f=w278) -> (s? t:f=w277:u32)
                  n141 = call "Loop Timer6"("Count(Ticks)"=w273) -> ()  [unwired: 1 out]
                  n142 = local read "Start Waveforms"() -> (w271:bool)
                  n143 = xnode "FPGA I/O Node"("Connector0/AO6"=w274) -> ()  [unwired: 1 in, 1 out]
                }
                n144 = node-c288(w265) -> ()
              }
              frame 4 {
                n145 = node-c288() -> (w301:T4)  [unwired: 1 in]
                n146 = timed-loop {
                  timing: w301 -> [_]
                  timing-out: [_] -> w300
                  tunnel: w305 -> [w309]
                  shift-right: [w307] -> _
                  shift-left: FALSE -> [w318]
                  shift-right: [w315] -> _
                  shift-left: _ -> [w314]
                  shift-right: [w312] -> _
                  shift-left: 0 -> [w310]
                  tunnel: w304 -> [w311]
                  tunnel: [w309] -> w302
                  stop <- w308 stop-if-true
                  n147 = Equal?(x=w311, y=w310) -> (x = y?=w308:bool)
                  n148 = xnode ("Register Read")() -> ("Data"=w307:bool)  [unwired: 1 in, 1 out]
                  n149 = Increment(x=w310) -> (x+1=w313:i32)
                  n150 = Greater?(x=w307, y=w318) -> (0:w316:bool)
                  n151 = Exclusive Or(1:w308, 2:w316) -> (0:w317:bool)
                  n152 = Select(t=w316, s=w317, f=w314) -> (s? t:f=w315:bool)
                  n153 = Select(t=w313, s=w314, f=w310) -> (s? t:f=w312:i32)
                }
                n154 = while {
                  shift-right: [w324] -> _
                  shift-left: w306 -> [w330]
                  tunnel: w303 -> [w332]
                  tunnel: w302 -> [w328]
                  tunnel: w306 -> [w327]
                  stop <- w326 continue-if-true
                  n155 = Increment(x=w330) -> (x+1=w333:u32)
                  n156 = Equal?(x=w330, y=w332) -> (x = y?=w331:bool)
                  n157 = xnode ("Memory Read")("Address"=w330) -> ("Data"=w329:i16)  [unwired: 1 in, 1 out]
                  n158 = Select(t=w327, s=w331, f=w333) -> (s? t:f=w324:u32)
                  n159 = call "Loop Timer13"("Count(Ticks)"=w328) -> ()  [unwired: 1 out]
                  n160 = Less?(x=w324, y=u32 4) -> (x < y?=w323:bool)
                  n161 = local write "Frame Trigger"(w323) -> ()
                  n162 = local read "Start Waveforms"() -> (w326:bool)
                  n163 = xnode "FPGA I/O Node"("Connector0/AO3"=w329) -> ()  [unwired: 1 in, 1 out]
                }
                n164 = node-c288(w300) -> ()
              }
              frame 5 {
                n165 = node-c288() -> (w340:T4)  [unwired: 1 in]
                n166 = node-c288() -> (w338:T4)  [unwired: 1 in]
                n167 = timed-loop {
                  timing: w340 -> [_]
                  timing-out: [_] -> w339
                  tunnel: w346 -> [w369]
                  tunnel: w344 -> [w368]
                  tunnel: [w368] -> w335
                  i -> [w371]
                  stop <- w370 stop-if-true
                  n168 = Equal?(x=w369, y=w371) -> (x = y?=w370:bool)
                }
                n169 = while {
                  shift-right: [w388] -> _
                  shift-left: w344 -> [w393]
                  tunnel: w348 -> [w394]
                  tunnel: w347 -> [w391]
                  tunnel: w344 -> [w390]
                  stop <- w386 continue-if-true
                  n170 = Increment(x=w393) -> (x+1=w395:u32)
                  n171 = Equal?(x=w393, y=w394) -> (x = y?=w389:bool)
                  n172 = call "Loop Timer14"("Count(Ticks)"=w391) -> ()  [unwired: 1 out]
                  n173 = xnode ("Memory Read")("Address"=w393) -> ("Data"=w392:i16)  [unwired: 1 in, 1 out]
                  n174 = Select(t=w390, s=w389, f=w395) -> (s? t:f=w388:u32)
                  n175 = Less?(x=w388, y=u32 20) -> (x < y?=w385:bool)
                  n176 = xnode ("Register Write")("Data"=w385) -> ()  [unwired: 1 in, 1 out]
                  n177 = local read "Start Waveforms"() -> (w386:bool)
                  n178 = xnode "FPGA I/O Node"("Connector0/AO5"=w392) -> ()  [unwired: 1 in, 1 out]
                }
                n179 = while {
                  shift-right: [w383] -> _
                  shift-left: w335 -> [w380]
                  tunnel: w345 -> [w382]
                  tunnel: w335 -> [w378]
                  tunnel: w343 -> [w377]
                  stop <- w376 continue-if-true
                  n180 = Increment(x=w380) -> (x+1=w384:u32)
                  n181 = Equal?(x=w380, y=w382) -> (x = y?=w381:bool)
                  n182 = xnode ("Memory Read")("Address"=w380) -> ("Data"=w379:i16)  [unwired: 1 in, 1 out]
                  n183 = Select(t=w378, s=w381, f=w384) -> (s? t:f=w383:u32)
                  n184 = call "Loop Timer16"("Count(Ticks)"=w377) -> ()  [unwired: 1 out]
                  n185 = local read "Start Waveforms"() -> (w376:bool)
                  n186 = xnode "FPGA I/O Node"("Connector0/AO6"=w379) -> ()  [unwired: 1 in, 1 out]
                }
                n187 = timed-loop {
                  timing: w338 -> [_]
                  timing-out: [_] -> w337
                  tunnel: w334 -> [w360]
                  tunnel: [w360] -> w336
                  tunnel: w341 -> [w361]
                  i -> [w363]
                  stop <- w362 stop-if-true
                  n188 = Equal?(x=w361, y=w363) -> (x = y?=w362:bool)
                }
                n189 = while {
                  shift-right: [w351] -> _
                  shift-left: w335 -> [w356]
                  tunnel: w342 -> [w358]
                  tunnel: w336 -> [w354]
                  tunnel: w335 -> [w353]
                  stop <- w352 continue-if-true
                  n190 = Increment(x=w356) -> (x+1=w359:u32)
                  n191 = Equal?(x=w356, y=w358) -> (x = y?=w357:bool)
                  n192 = xnode ("Memory Read")("Address"=w356) -> ("Data"=w355:i16)  [unwired: 1 in, 1 out]
                  n193 = Select(t=w353, s=w357, f=w359) -> (s? t:f=w351:u32)
                  n194 = Less?(x=w351, y=u32 4) -> (x < y?=w349:bool)
                  n195 = local write "Frame Trigger"(w349) -> ()
                  n196 = call "Loop Timer18"("Count(Ticks)"=w354) -> ()  [unwired: 1 out]
                  n197 = xnode "FPGA I/O Node"("Connector0/AO3"=w355) -> ()  [unwired: 1 in, 1 out]
                  n198 = local read "Start Waveforms"() -> (w352:bool)
                }
                n199 = node-c288(w339) -> ()
                n200 = node-c288(w337) -> ()
              }
              frame 6 {
                n201 = node-c288() -> (w406:T4)  [unwired: 1 in]
                n202 = while {
                  tunnel: w403 -> [_]
                  tunnel: w402 -> [w422]
                  tunnel: w399 -> [w423]
                  tunnel: w401 -> [w426]
                  tunnel: w396 -> [w428]
                  stop <- w429 continue-if-true
                  n203 = Quotient & Remainder(x="Current Frame", y=w426) -> (x-y*floor(x/y)=w421:u8)  [unwired: 1 out]
                  n204 = To Word Integer(number=w421) -> (16bit integer=w420:i16)
                  n205 = call "Loop Timer21"("Count(Ticks)"=w428) -> ()  [unwired: 1 out]
                  n206 = Multiply(x=w422, y=w420) -> (x*y=w425:i16)
                  n207 = Add(x=w425, y=w423) -> (x+y=w424:i16)
                  n208 = local read "Start Waveforms"() -> (w429:bool)
                  n209 = xnode "FPGA I/O Node"("Connector0/AO3"=w424) -> ()  [unwired: 1 in, 1 out]
                }
                n210 = while {
                  tunnel: w398 -> [w419]
                  tunnel: w404 -> [w418]
                  tunnel: w396 -> [w417]
                  shift-right: [w415] -> _
                  shift-left: w398 -> [w416]
                  stop <- w409 continue-if-true
                  n211 = Increment(x=w416) -> (x+1=w414:u32)
                  n212 = Equal?(x=w416, y=w418) -> (x = y?=w412:bool)
                  n213 = xnode ("Memory Read")("Address"=w416) -> ("Data"=w413:i16)  [unwired: 1 in, 1 out]
                  n214 = Select(t=w419, s=w412, f=w414) -> (s? t:f=w415:u32)
                  n215 = call "Loop Timer19"("Count(Ticks)"=w417) -> ()  [unwired: 1 out]
                  n216 = Less?(x=w415, y=u32 4) -> (x < y?=w410:bool)
                  n217 = local write "Frame Trigger"(w410) -> ()
                  n218 = xnode "FPGA I/O Node"("Connector0/AO5"=w413) -> ()  [unwired: 1 in, 1 out]
                  n219 = local read "Start Waveforms"() -> (w409:bool)
                }
                n220 = timed-loop {
                  timing: w406 -> [_]
                  timing-out: [_] -> w405
                  tunnel: w396 -> [w441]
                  tunnel: [w441] -> w397
                  tunnel: w407 -> [w442]
                  i -> [w444]
                  stop <- w443 stop-if-true
                  n221 = Equal?(x=w442, y=w444) -> (x = y?=w443:bool)
                }
                n222 = while {
                  shift-right: [w432] -> _
                  shift-left: w398 -> [w438]
                  tunnel: w408 -> [w439]
                  tunnel: w397 -> [w436]
                  tunnel: w398 -> [w435]
                  tunnel: w400 -> [w431]
                  stop <- w434 continue-if-true
                  n223 = Increment(x=w438) -> (x+1=w440:u32)
                  n224 = Equal?(x=w438, y=w439) -> (x = y?=w433:bool)
                  n225 = xnode ("Memory Read")("Address"=w438) -> ("Data"=w437:i16)  [unwired: 1 in, 1 out]
                  n226 = Select(t=w435, s=w433, f=w440) -> (s? t:f=w432:u32)
                  n227 = Greater?(x=w431, y=w432) -> (0:→"End Linear Ramp":bool)
                  n228 = call "Loop Timer20"("Count(Ticks)"=w436) -> ()  [unwired: 1 out]
                  n229 = local read "Start Waveforms"() -> (w434:bool)
                  n230 = xnode "FPGA I/O Node"("Connector0/AO6"=w437) -> ()  [unwired: 1 in, 1 out]
                }
                n231 = node-c288(w405) -> ()
              }
              frame 7 {
                w458 = u8 0
                n232 = node-c288() -> (w463:T4)  [unwired: 1 in]
                n233 = while {
                  shift-right: [w511] -> _
                  shift-left: w464 -> [w517]
                  tunnel: w451 -> [w518]
                  tunnel: w452 -> [w515]
                  tunnel: w464 -> [w514]
                  stop <- w513 continue-if-true
                  n234 = Increment(x=w517) -> (x+1=w519:u32)
                  n235 = Equal?(x=w517, y=w518) -> (x = y?=w512:bool)
                  n236 = xnode ("Memory Read")("Address"=w517) -> ("Data"=w516:i16)  [unwired: 1 in, 1 out]
                  n237 = Select(t=w514, s=w512, f=w519) -> (s? t:f=w511:u32)
                  n238 = call "Loop Timer4"("Count(Ticks)"=w515) -> ()  [unwired: 1 out]
                  n239 = Less?(x=w511, y=u32 20) -> (x < y?=w509:bool)
                  n240 = xnode "FPGA I/O Node"("TRIG0"=w509) -> ()  [unwired: 1 in, 1 out]
                  n241 = local read "Start Waveforms"() -> (w513:bool)
                  n242 = xnode "FPGA I/O Node"("Connector0/AO1"=w516) -> ()  [unwired: 1 in, 1 out]
                }
                n243 = while {
                  shift-right: [w465] -> _
                  shift-left: FALSE -> [w488]
                  shift-right: [w482] -> _
                  shift-left: w458 -> [w484]
                  tunnel: w460 -> [w483]
                  shift-right: [w466] -> _
                  shift-left: w456 -> [w479]
                  tunnel: w459 -> [w478]
                  shift-right: [w472] -> _
                  shift-left: w458 -> [w475]
                  tunnel: w457 -> [w471]
                  tunnel: w456 -> [w468]
                  tunnel: w453 -> [w467]
                  stop <- w489 continue-if-true
                  n244 = local read "End Linear Ramp"() -> (w465:bool)
                  n245 = Increment(x=w484) -> (x+1=w487:u8)
                  n246 = Greater?(x=w465, y=w488) -> (0:w486:bool)
                  n247 = Select(t=w487, s=w486, f=w484) -> (s? t:f=w481:u8)
                  n248 = Add(x=w478, y=w479) -> (x+y=w480:i16)
                  n249 = Increment(x=w475) -> (x+1=w476:u8)
                  n250 = Equal?(x=w481, y=w483) -> (x = y?=w477:bool)
                  n251 = Select(t=u8 0, s=w477, f=w481) -> (s? t:f=w482:u8)
                  n252 = Select(t=w476, s=w477, f=w475) -> (s? t:f=w473:u8)
                  n253 = Select(t=w480, s=w477, f=w479) -> (s? t:f=w474:i16)
                  n254 = call "Loop Timer17"("Count(Ticks)"=w467) -> ()  [unwired: 1 out]
                  n255 = Equal?(x=w473, y=w471) -> (x = y?=w470:bool)
                  n256 = local read "Start Waveforms"() -> (w489:bool)
                  n257 = Select(t=w468, s=w470, f=w474) -> (s? t:f=w466:i16)
                  n258 = xnode "FPGA I/O Node"("Connector0/AO3"=w466) -> ()  [unwired: 1 in, 1 out]
                  n259 = Select(t=u8 0, s=w470, f=w473) -> (s? t:f=w472:u8)
                }
                n260 = timed-loop {
                  timing: w463 -> [_]
                  timing-out: [_] -> w462
                  tunnel: w453 -> [w501]
                  tunnel: [w501] -> w454
                  tunnel: w450 -> [w502]
                  i -> [w504]
                  stop <- w503 stop-if-true
                  n261 = Equal?(x=w502, y=w504) -> (x = y?=w503:bool)
                }
                n262 = while {
                  shift-right: [w492] -> _
                  shift-left: w464 -> [w498]
                  tunnel: w449 -> [w499]
                  tunnel: w454 -> [w496]
                  tunnel: w464 -> [w495]
                  tunnel: w455 -> [w491]
                  stop <- w494 continue-if-true
                  n263 = Increment(x=w498) -> (x+1=w500:u32)
                  n264 = Equal?(x=w498, y=w499) -> (x = y?=w493:bool)
                  n265 = xnode ("Memory Read")("Address"=w498) -> ("Data"=w497:i16)  [unwired: 1 in, 1 out]
                  n266 = Select(t=w495, s=w493, f=w500) -> (s? t:f=w492:u32)
                  n267 = Greater?(x=w491, y=w492) -> (0:w490:bool)
                  n268 = local write "End Linear Ramp"(w490) -> ()
                  n269 = call "Loop Timer15"("Count(Ticks)"=w496) -> ()  [unwired: 1 out]
                  n270 = local read "Start Waveforms"() -> (w494:bool)
                  n271 = xnode "FPGA I/O Node"("Connector0/AO2"=w497) -> ()  [unwired: 1 in, 1 out]
                }
                n272 = node-c288(w462) -> ()
              }
            }
            n273 = case shown="3" w80 {
              frame 0, Default {
              }
              frame 3 {
                n274 = while {
                  stop <- w141 continue-if-true
                  n275 = local read "Start Waveforms"() -> (w141:bool)
                  n276 = xnode "FPGA I/O Node"("Connector0/AO1"="X Piezo Axis", "Connector0/AO2"="Y Piezo Axis", "Connector0/AO3"="Z Piezo Axis") -> ()  [unwired: 3 in, 3 out]
                }
              }
            }
            n277 = Index Array(array="Accums Per Line", index #1=0 ("index"), index #2=1 ("index"), index #3=2 ("index"), index #4=3 ("index")) -> (element #1=w86:u32, element #2=w85:u32, element #3=w84:u32, element #4=w83:u32)
            n278 = Compound Arithmetic op=ADD(w86, w85, w84, w83) -> (w93:u32)
            n279 = Multiply(x="Number of Lines", y=w93) -> (x*y=w94:u32)
            n280 = node-c288() -> (w96:T4)  [unwired: 1 in]
            n281 = timed-loop {
              timing: w96 -> [_]
              timing-out: [_] -> w95
              shift-right: [w130] -> _
              shift-left: w82 -> [w110]
              shift-right: [w128] -> _
              shift-left: _ -> [w111]
              shift-right: [w129] -> _
              shift-left: _ -> [w127]
              shift-right: [w114] -> _
              shift-left: u32 0 -> [w119]
              shift-right: [w123] -> _
              shift-left: w82 -> [w121]
              tunnel: w94 -> [w118]
              tunnel: w80 -> [w112]
              stop <- "Stop Sync Signal" continue-if-true
              n282 = Increment(x=w119) -> (x+1=w122:u32)
              n283 = Equal?(x=w119, y=w118) -> (x = y?=w116:bool)
              n284 = And(x=w111, y=w121) -> (x .and. y?=w126:bool)
              n285 = And(x=w121, y=w111) -> (x .and. y?=w120:bool)
              n286 = local read "Frame Trigger"() -> (w125:bool)
              n287 = Select(t=w122, s=w120, f=w119) -> (s? t:f=w117:u32)
              n288 = case shown="True" w127 {
                tunnel: w126 -> [_ w133]
                frame False {
                }
                frame True {
                  n289 = xnode "FPGA I/O Node"("TRIG1"=w133) -> ()  [unwired: 1 in, 1 out]
                  "Laser Blank Trigger" <- w133
                }
              }
              n290 = xnode ("Register Write")("Data"=w110) -> ()  [unwired: 1 in, 1 out]
              n291 = case shown="0, Default" w112 {
                tunnel: [w131 w132] -> w130
                frame 0, Default {
                  n292 = xnode "FPGA I/O Node"() -> ("Connector1/DIO0"=w131:bool)  [unwired: 1 in, 1 out]
                }
                frame 5 {
                  n293 = xnode ("Register Read")() -> ("Data"=w132:bool)  [unwired: 1 in, 1 out]
                }
              }
              n294 = Exclusive Or(1:w116, 2:w125) -> (0:w124:bool)
              n295 = Select(t=w125, s=w124, f=w121) -> (s? t:f=w123:bool)
              n296 = Select(t=u32 0, s=w116, f=w117) -> (s? t:f=w114:u32)
              n297 = Not Equal?(x=w130, y=w110) -> (x != y?=w129:bool)
              n298 = Greater?(x=w130, y=w110) -> (0:w128:bool)
            }
            n299 = node-c288(w95) -> ()
          }
        }
      }
    }
    n300 = xnode "FPGA I/O Node"("Connector0/AO0"=i16 0) -> ()  [unwired: 1 in, 1 out]
  }
  n301 = local read "Accums Per Line"() -> (w1:u32[])
  n302 = while {
    shift-right: [w563] -> _
    shift-left: u8 0 -> [w540]
    shift-right: [w564] -> _
    shift-left: w2 -> [w568]
    shift-right: [w562] -> _
    shift-left: u8 0 -> [w565]
    tunnel: "Sequences" -> [w561]
    shift-right: [w555] -> _
    shift-left: u32 0 -> [w556]
    tunnel: w1 -> [w542]
    shift-right: [w522] -> _
    shift-left: w2 -> [w537]
    stop <- FALSE stop-if-true
    n303 = local read "Laser Blank Trigger"() -> (w522:bool)
    n304 = To Long Integer(number=w540) -> (32bit integer=w539:i32)
    n305 = Add(x="Laser Delay (Ticks)", y="Laser On Time (Ticks)") -> (x+y=w526:u8)
    n306 = Index Array(array=w542, index=w539) -> (element=w541:u32)
    n307 = Increment(x=w556) -> (x+1=w557:u32)
    n308 = Equal?(x=w556, y=w541) -> (x = y?=w553:bool)
    n309 = Equal?(x=w565, y=w526) -> (x = y?=w554:bool)
    n310 = Greater?(x=w522, y=w537) -> (0:w536:bool)
    n311 = Select(t=w557, s=w554, f=w556) -> (s? t:f=w558:u32)
    n312 = Increment(x=w540) -> (x+1=w573:u8)
    n313 = Equal?(x=w540, y=w561) -> (x = y?=w570:bool)
    n314 = Exclusive Or(1:w554, 2:w536) -> (0:w569:bool)
    n315 = Select(t=u32 0, s=w553, f=w558) -> (s? t:f=w555:u32)
    n316 = Select(t=w573, s=w553, f=w540) -> (s? t:f=w572:u8)
    n317 = Increment(x=w565) -> (x+1=w567:u8)
    n318 = Select(t=w536, s=w569, f=w568) -> (s? t:f=w564:bool)
    n319 = Split Number(x="Laser States") -> (hi(x)=w550:u16, lo(x)=w551:u16)
    n320 = Select(t=u8 0, s=w570, f=w572) -> (s? t:f=w563:u8)
    n321 = Select(t=w567, s=w564, f=u8 0) -> (s? t:f=w562:u8)
    n322 = Split Number(x=w550) -> (hi(x)=w549:u8, lo(x)=w548:u8)
    n323 = Split Number(x=w551) -> (hi(x)=w547:u8, lo(x)=w546:u8)
    n324 = Greater?(x=w562, y="Laser Delay (Ticks)") -> (0:w538:bool)
    n325 = call "Loop Timer22"("Count(Ticks)"=u16 80) -> ()  [unwired: 1 out]
    n326 = case shown="0, Default" w563 {
      tunnel: w549 -> [w574 _ _ _]
      tunnel: w548 -> [_ w575 _ _]
      tunnel: w547 -> [_ _ w576 _]
      tunnel: w546 -> [_ _ _ w577]
      tunnel: [w574 w575 w576 w577] -> w545
      frame 0, Default {
      }
      frame 1 {
      }
      frame 2 {
      }
      frame 3 {
      }
    }
    n327 = Or(x="Blanking Off/Manual", y=w538) -> (x .or. y?=w521:bool)
    n328 = Select(t=w545, s=w521, f=u8 0) -> (s? t:f=w533:u8)
    n329 = Number To Boolean Array(number=w533) -> (Boolean array=w535:bool[])
    n330 = xnode "FPGA I/O Node"("Connector1/DIO4"="Blanking Off/Manual") -> ()  [unwired: 1 in, 1 out]
    n331 = Index Array(array=w535, index #1=0 ("index"), index #2=1 ("index"), index #3=2 ("index"), index #4=3 ("index")) -> (element #1=w529:bool, element #2=w528:bool, element #3=w524:bool, element #4=w523:bool)
    n332 = xnode "FPGA I/O Node"("Connector0/DIO0"=w529, "Connector1/DIO8"=w528, "Connector1/DIO9"=w524, "Connector1/DIO10"=w523) -> ()  [unwired: 4 in, 4 out]
  }
  n333 = while {
    stop <- "stop" stop-if-true
    n334 = call "Loop Timer23"("Count(uSec)"=u32 100) -> ()  [unwired: 1 out]
    n335 = xnode "FPGA I/O Node"("Connector1/DIO26"="Lower Shutter Command", "Connector1/DIO28"="Upper Shutter Command") -> ("Connector1/DIO25"=→"Lower Shutter Status":bool, "Connector1/DIO27"=→"Upper Shutter Status":bool)  [unwired: 4 in, 4 out]
  }
